vi "Start AC Source.vi"(7 "AC sync source":T1, 8 "error in (no error)":errorcluster, 9 "Signal amplitude (V)":dbl, 10 "Signal frequency  (Hz)":dbl, 11 "AC source":T1) -> (0 "error out":errorcluster, 2 "status":string, 3 "AC source out":T1, 5 "AC sync source out":T1)   [LabVIEW 2020]
doc: "Set required values and properties to the AC source and switch it on."
uses:
  Type definitions/AC Source.ctl
  Type definitions/AC Source type.ctl
  <vilib>/Utility/error.llb/Error Cluster From Error Code.vi
  <vilib>/ErrorRing/Error Ring.xnode
  external libraries/Fluke 5XXX Series Multicalibrator/Fluke 5XXX Series Multicalibrators.lvlib
  external libraries/AWG/AFG3000/Tektronix AFG 3000 Series.lvlib
  external libraries/varilib/varilib.lvlib
  external libraries/AWG/Agilent 33XXX Series/Agilent 33XXX Series.lvlib
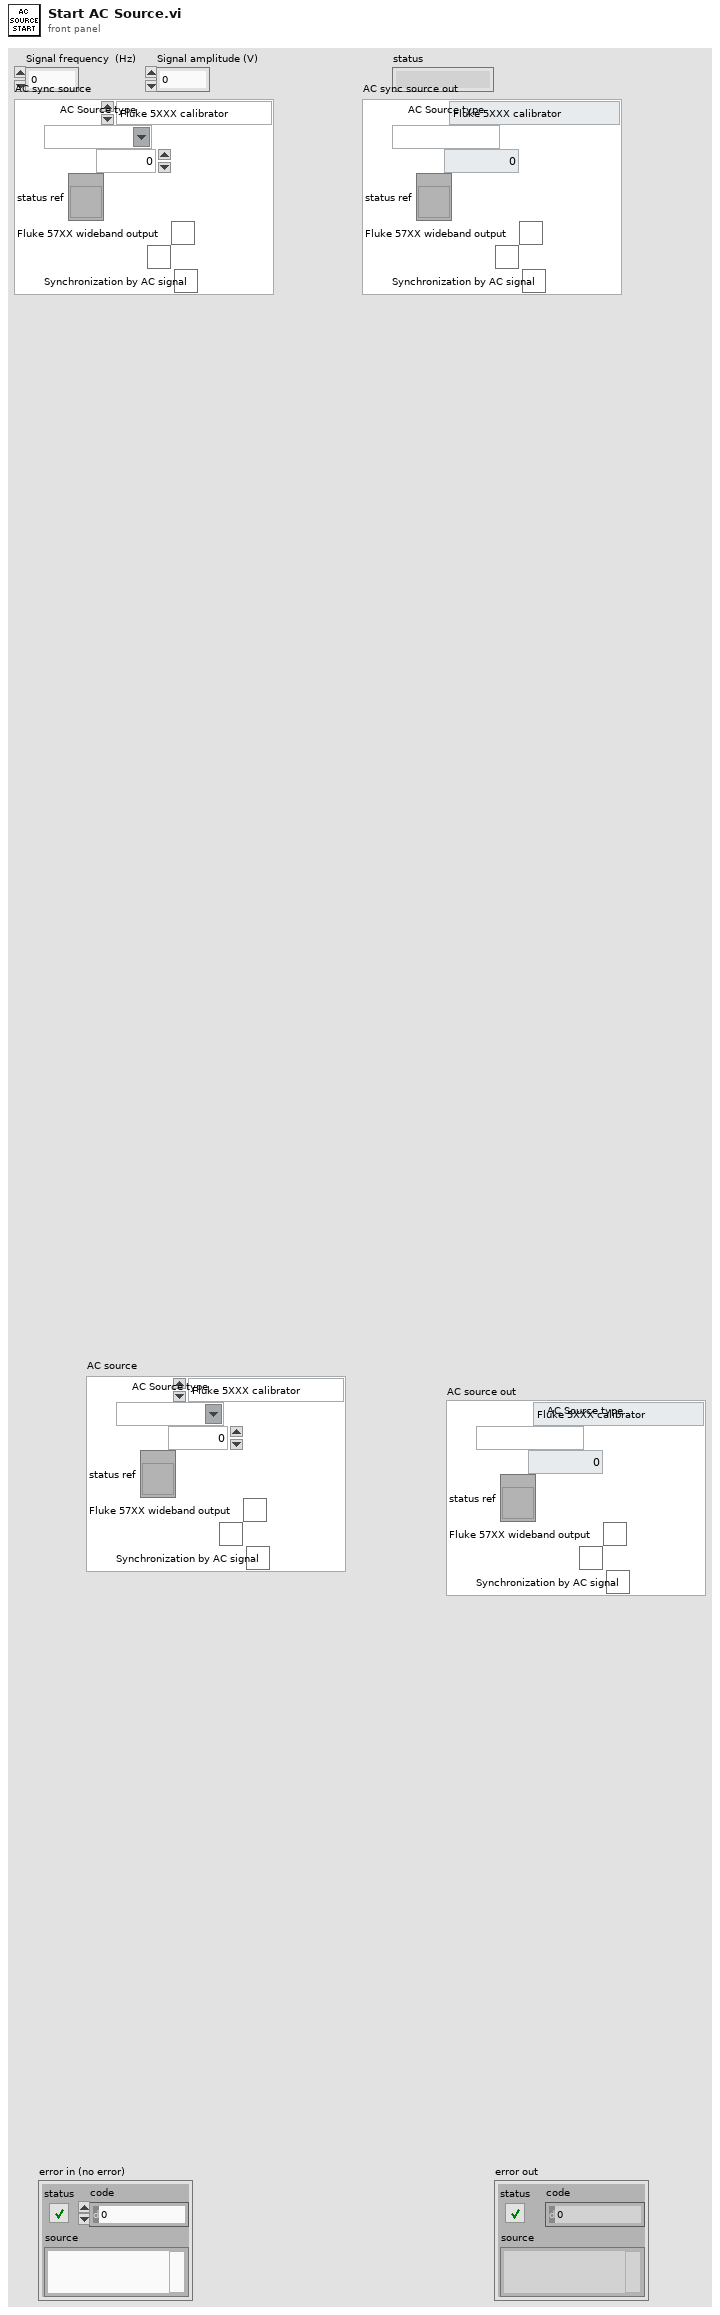
[diagram p1: front panel]
types:
  T1 = typedef "AC Source.ctl" = cluster{"AC Source type":T2, "VISA":refnum<visa-resource-name>, "Ref. clock (Hz)":dbl, "status ref":refnum<vi>, "Fluke 57XX wideband output":bool, "Fluke 57XX ignore errors":bool, "Synchronization by AC signal":bool}
  T2 = typedef "AC Source type.ctl" = enum16{"Fluke 5XXX calibrator", "Tektronix AFG3000 series", "dummy", "Agilent 331xxA to 332xxA", "Agilent 335xxA to 336xxA"}
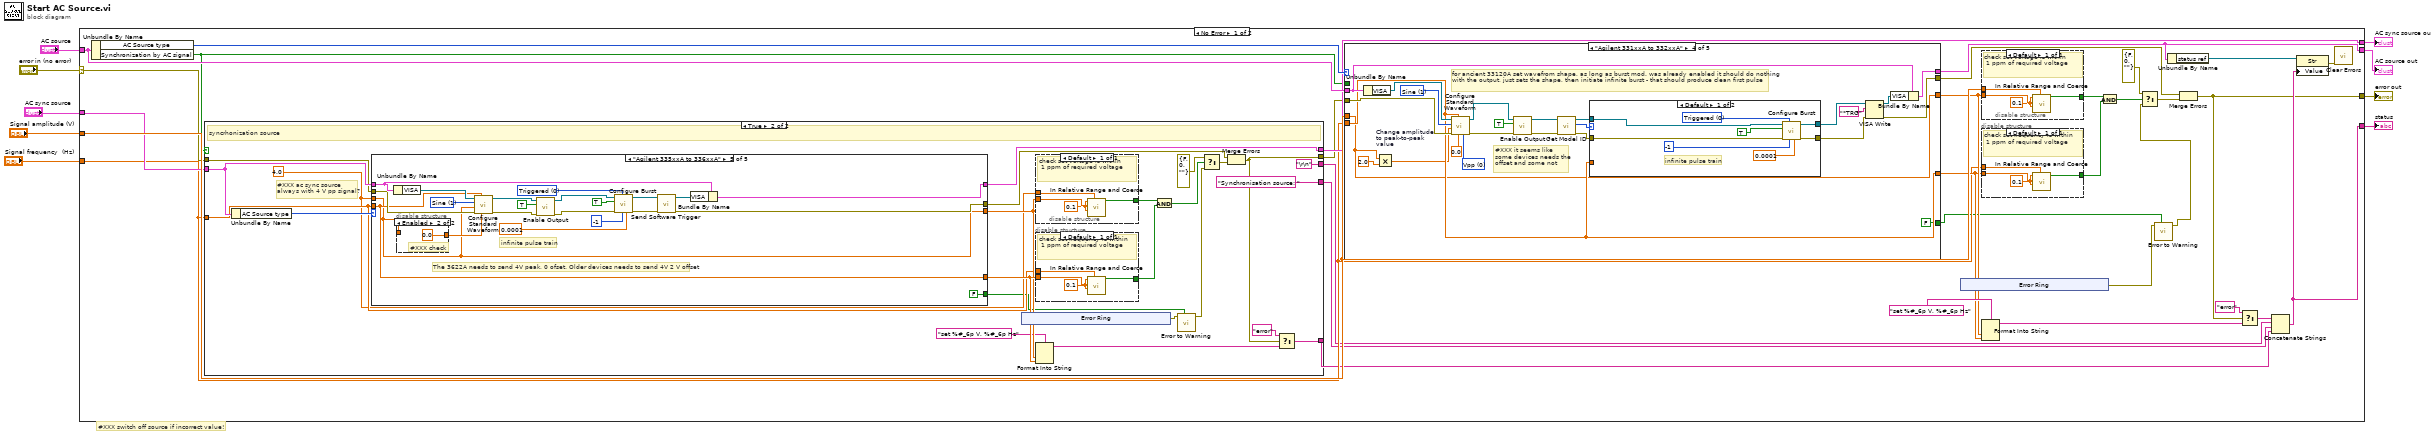
[diagram p0: block diagram]
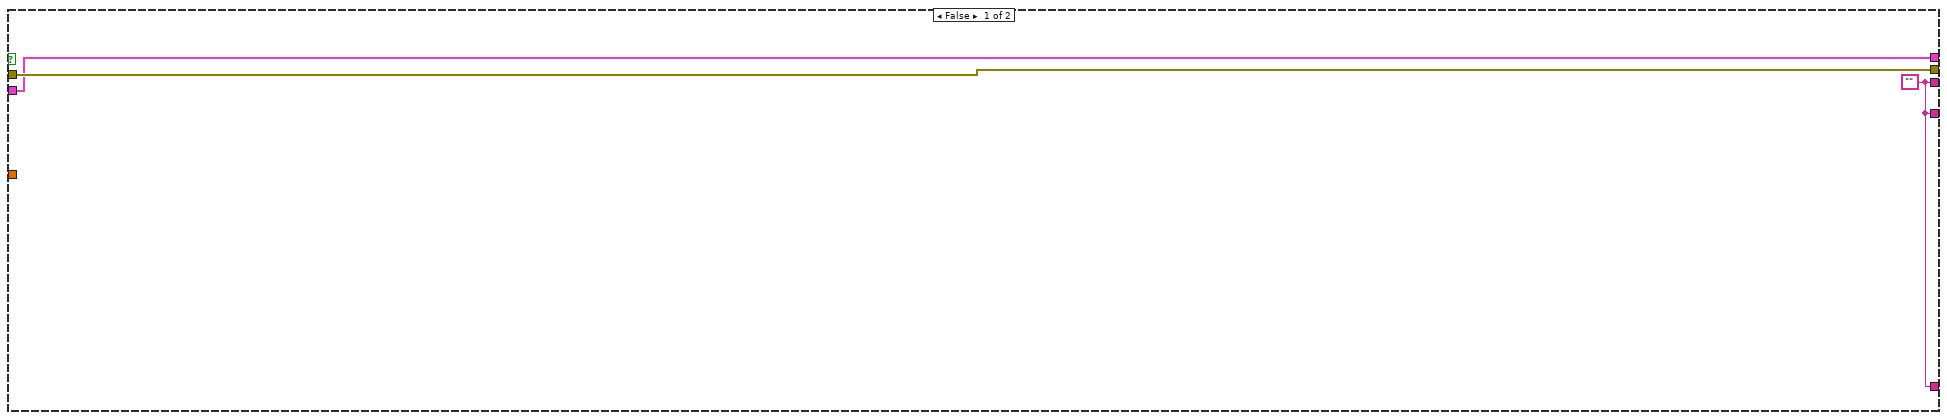
[diagram p2: hidden frame]
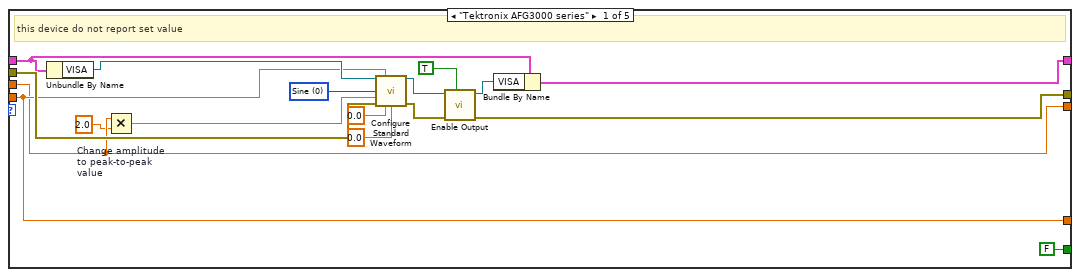
[diagram p3: hidden frame]
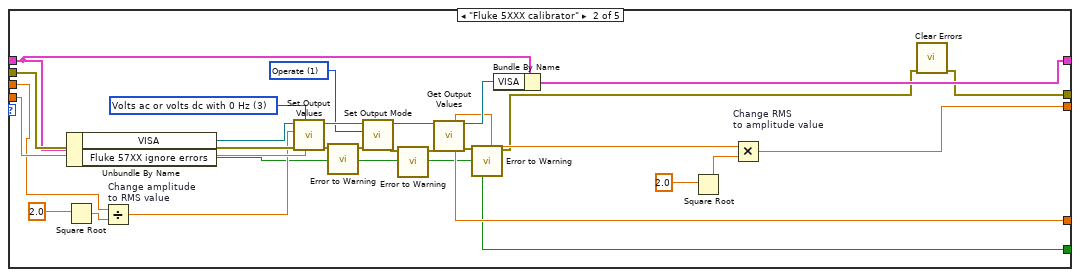
[diagram p4: hidden frame]
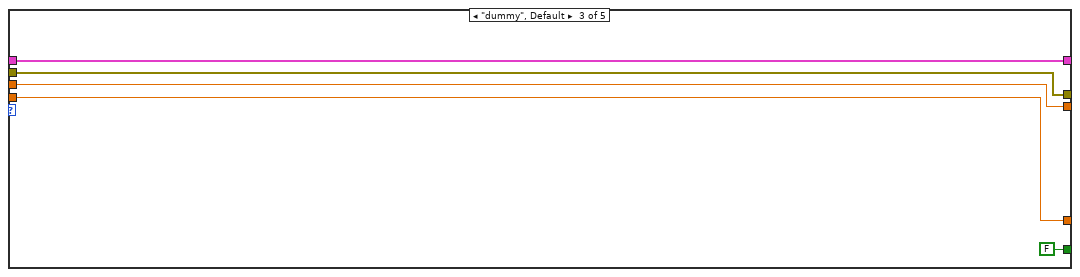
[diagram p5: hidden frame]
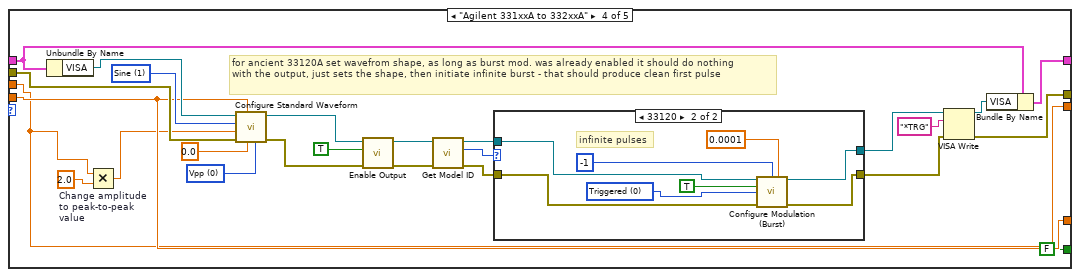
[diagram p6: hidden frame]
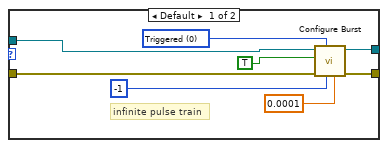
[diagram p7: hidden frame]
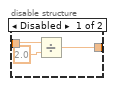
[diagram p8: hidden frame]
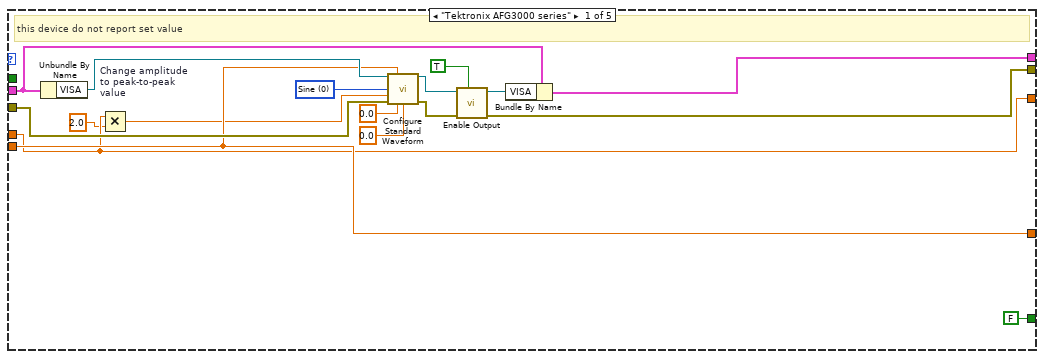
[diagram p9: hidden frame]
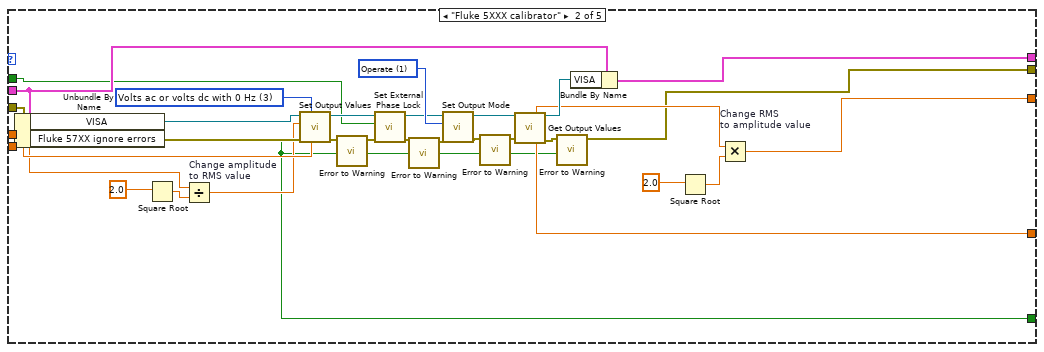
[diagram p10: hidden frame]
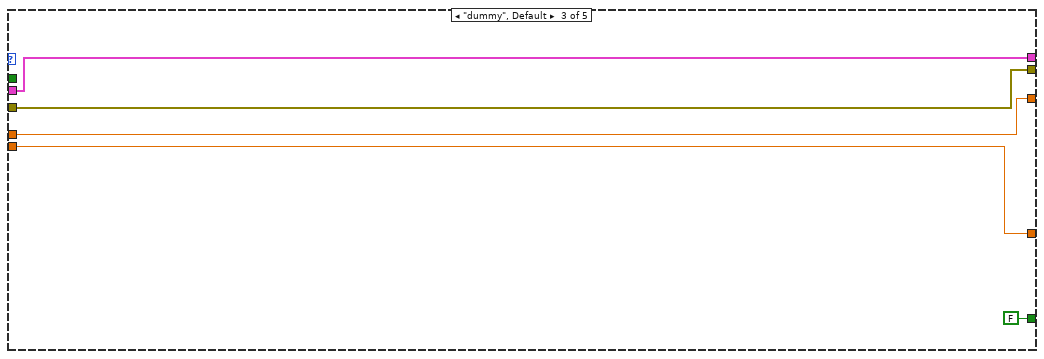
[diagram p11: hidden frame]
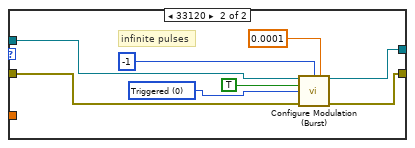
[diagram p12: hidden frame]
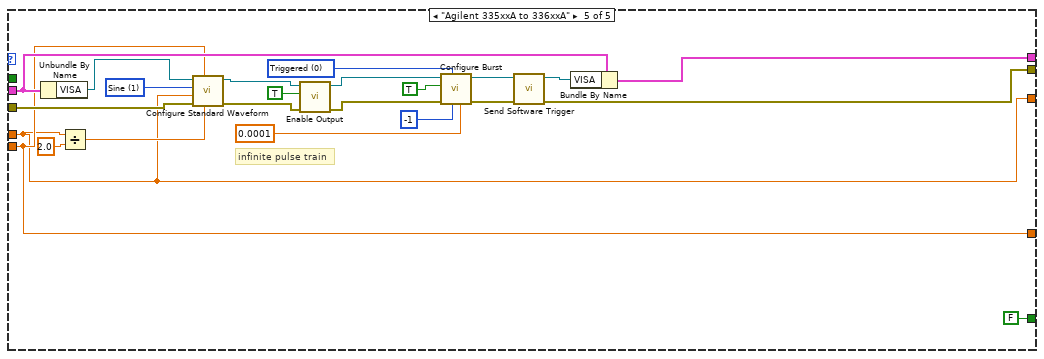
[diagram p13: hidden frame]
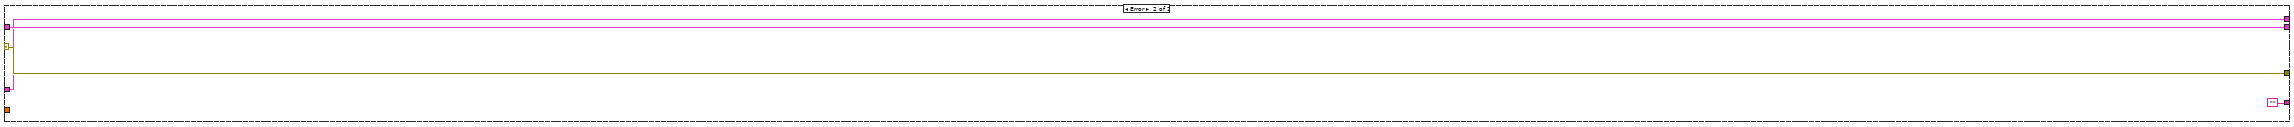
[diagram p14: hidden frame]
diagram:
  # "#XXX switch off source if incorrect value!"
  n1 = case shown="No Error" "error in (no error)" {
    selector: "error in (no error)" -> [w15 w330]
    tunnel: "AC source" -> [w40 w328]
    tunnel: "Signal frequency  (Hz)" -> [w20 _]
    tunnel: "Signal amplitude (V)" -> [w37 _]
    tunnel: [w14 w330] -> w7
    tunnel: [w21 ""] -> w6
    tunnel: [w25 w328] -> w4
    tunnel: "AC sync source" -> [w24 w327]
    tunnel: [w23 w327] -> w2
    frame No Error {
      n2 = Unbundle By Name(w40) -> ("AC Source type"=w41:T2, "Synchronization by AC signal"=w16:bool)
      n3 = case shown="True" w16 {
        tunnel: w15 -> [w44 w57]
        tunnel: [w44 w48] -> w13
        tunnel: w24 -> [w43 w58]
        tunnel: [w43 w56] -> w23
        tunnel: w20 -> [_ w50]
        tunnel: [w42 "\r\n"] -> w19
        tunnel: [w42 "Synchronisation source: " ("string")] -> w18
        tunnel: [w42 w51] -> w17
        frame False {
          w42 = ""
        }
        frame True {
          w49 = 4.0 ("Signal frequency  (Hz)")
          # "#XXX ac sync source\nalways with 4 V pp signal?"
          # "syncrhonization source"
          n4 = Unbundle By Name(w58) -> ("AC Source type"=w59:T2)
          n5 = case shown="\"Agilent 335xxA to 336xxA\"" w59 {
            tunnel: w57 -> [w95 w125 w129 w146 w179]
            tunnel: [w87 w106 w129 w138 w177] -> w66
            tunnel: w58 -> [w93 w124 w130 w144 w181]
            tunnel: [w92 w123 w130 w143 w180] -> w56
            tunnel: w50 -> [w86 w115 w127 w137 w174]
            tunnel: w49 -> [w85 w112 w128 w132 w173]
            tunnel: [w85 w107 w128 w132 w173] -> w63
            tunnel: [w86 w116 w127 w137 w174] -> w64
            tunnel: [FALSE ("Fluke 57XX ignore errors") w99 FALSE ("Fluke 57XX ignore errors") FALSE ("Fluke 57XX ignore errors") FALSE ("Fluke 57XX ignore errors")] -> w45
            frame "Tektronix AFG3000 series" {
              w96 = u16 0 items=["Sine", "Square", "Pulse", "Ramp", "Noise", "DC", "Sin(x)/x", "Gaussian", "Lorentz", "Exponential Rise", "Exponential Decay", "Haversine"] ("Waveform Function (0: Sine)")
              # "this device do not report set value"
              n6 = Unbundle By Name(w93) -> ("VISA"=w94:refnum<visa-resource-name>)
              n7 = Multiply "Change amplitude\nto peak-to-peak\nvalue"(x=w85, y=2.0) -> (x*y=w83:dbl)
              n8 = call "Configure Standard Waveform.vi"("VISA resource name"=w94, "Frequency (1000 Hz)"=w86, "Waveform Function (0: Sine)"=w96, "Amplitude (1 Vpp)"=w83, "error in (no error)"=w95, "DC Offset (0.00 V)"=0.0, "Phase Level (-1)"=0.0) -> ("VISA resource name out"=w90:refnum<visa-resource-name>, "error out"=w88:errorcluster)  [unwired: 7 in]
              n9 = call "Enable Output.vi"("Enable Output (T: Enable)"=TRUE, "error in (no error)"=w88, "VISA resource name"=w90) -> ("error out"=w87:errorcluster, "VISA resource name out"=w89:refnum<visa-resource-name>)  [unwired: 7 in]
              n10 = Bundle By Name(cluster=w93, "VISA"=w89) -> (w92:T1)
            }
            frame "Fluke 5XXX calibrator" {
              w119 = u32 1 items=["Standby", "Operate"] ("Output Mode (0: Standby)")
              w121 = u32 3 items=["Amplitude", "Volts dc or update volts ac", "Volts ac dBm update", "Volts ac or volts dc with 0 Hz", "Volts ac in dBm", "Current dc or update current ac", "Current ac", "Update frequency", "Resistance", "Capacitance", "Temperature (Celsius)", "Temperature (Fahrenheit)", "Power dc or update power ac", "Power ac", "Dual volts dc or update dual ac", "Dual volts ac in volts", "Power ac in dBm update", "Power ac in dBm", "Dual volts ac in dBm update", "Dual volts ac in dBm"] ("Output Value(s) (0 - Amplitude)")
              n11 = Square Root(x=2.0 ("y")) -> (sqrt(x)=w113:dbl)
              n12 = Unbundle By Name(w124) -> ("VISA"=w122:refnum<visa-resource-name>, "Fluke 57XX ignore errors"=w99:bool)
              n13 = Divide "Change amplitude\nto RMS value"(x=w112, y=w113) -> (x/y=w111:dbl)
              n14 = call "Set Output Values.vi"("Fundamental Frequency (0.0 Hz)"=w115, "Output Value(s) (0 - Amplitude)"=w121, "error in (no error)"=w125, "Primary Value (0.0)"=w111, "VISA resource name"=w122) -> ("error out"=w105:errorcluster, "VISA resource name out"=w120:refnum<visa-resource-name>)  [unwired: 5 in]
              n15 = call "Error to Warning.vi"("Change to warning?"=w99, "error in (no error)"=w105) -> ("error out"=w104:errorcluster)  [unwired: 9 in]
              n16 = call "Set Output Mode.vi"("error in (no error)"=w104, "Output Mode (0: Standby)"=w119, "VISA resource name"=w120) -> ("error out"=w103:errorcluster, "VISA resource name out"=w118:refnum<visa-resource-name>)  [unwired: 7 in]
              n17 = call "Error to Warning.vi"("Change to warning?"=w99, "error in (no error)"=w103) -> ("error out"=w102:errorcluster)  [unwired: 9 in]
              n18 = call "Get Output Values.vi"("VISA resource name"=w118, "error in (no error)"=w102) -> ("Primary Value"=w108:dbl, "VISA resource name out"=w117:refnum<visa-resource-name>, "Fundamental Frequency"=w116:dbl, "error out"=w101:errorcluster)  [unwired: 7 in, 3 out]
              n19 = call "Error to Warning.vi"("Change to warning?"=w99, "error in (no error)"=w101) -> ("error out"=w100:errorcluster)  [unwired: 9 in]
              n20 = Bundle By Name(cluster=w124, "VISA"=w117) -> (w123:T1)
              n21 = Square Root(x=2.0 ("y")) -> (sqrt(x)=w110:dbl)
              n22 = Multiply "Change RMS\nto amplitude value"(x=w108, y=w110) -> (x*y=w107:dbl)
              n23 = call <vilib>:"Clear Errors.vi"("error in (no error)"=w100) -> ("error out"=w106:errorcluster)  [unwired: 5 in, 1 out]
            }
            frame "dummy", Default {
            }
            frame "Agilent 331xxA to 332xxA" {
              w136 = u16 0 items=["Vpp", "Vrms", "dB"] ("Unit (0: Vpp)")
              w155 = u16 1 items=["DC", "Sine", "Square", "Triangle", "Ramp", "Pulse", "Noise", "Sinc", "Negative Ramp", "Exponential Rise", "Exponential Fall", "Cardiac"] ("Waveform Function (1: Sine)")
              # "for ancient 33120A set wavefrom shape, as long as burst mod. was already enabled it should do nothing\nwith the output, just sets the shape, then initiate infinite burst - that should produce clean first pulse"
              n24 = Unbundle By Name(w144) -> ("VISA"=w145:refnum<visa-resource-name>)
              n25 = Multiply "Change amplitude\nto peak-to-peak\nvalue"(x=w132, y=2.0) -> (x*y=w131:dbl)
              n26 = call "Configure Standard Waveform.vi"("Unit (0: Vpp)"=w136, "DC Offset (0.00 V)"=0.0, "Frequency (1000 Hz)"=w137, "error in (no error)"=w146, "Amplitude (1)"=w131, "Waveform Function (1: Sine)"=w155, "VISA resource name"=w145) -> ("error out"=w154:errorcluster, "VISA resource name out"=w153:refnum<visa-resource-name>)  [unwired: 3 in]
              n27 = call "Enable Output.vi"("error in (no error)"=w154, "Enable Output  (T: Enable)"=TRUE, "VISA resource name"=w153) -> ("error out"=w151:errorcluster, "VISA resource name out"=w150:refnum<visa-resource-name>)  [unwired: 7 in]
              n28 = call "Get Model ID.vi"("error in (no error)"=w151, "VISA resource name"=w150) -> ("error out"=w149:errorcluster, "model ID"=w148:u32, "VISA resource name out"=w147:refnum<visa-resource-name>)  [unwired: 7 in]
              n29 = case shown="33120" w148 {
                tunnel: [w162 w168] -> w139
                tunnel: [w161 w167] -> w141
                tunnel: w149 -> [w163 w166]
                tunnel: w147 -> [w160 w165]
                frame Default {
                  w159 = u16 0 items=["Triggered", "Gated"] ("Burst Mode (0: Triggered)")
                  # "infinite pulse train"
                  n30 = call "Configure Burst.vi"("Burst Period (1 s)"=0.0001, "Burst Count (1)"=-1, "Burst Mode (0: Triggered)"=w159, "error in (no error)"=w163, "Enable Burst (T: Enable)"=TRUE, "VISA resource name"=w160) -> ("error out"=w162:errorcluster, "VISA resource name out"=w161:refnum<visa-resource-name>)  [unwired: 4 in]
                }
                frame 33120 {
                  w169 = u16 0 items=["Triggered", "Gated"] ("Burst Modulation Mode (0: Triggered)")
                  # "infinite pulses"
                  n31 = call "Configure Modulation (Burst).vi"("VISA resource name"=w165, "Burst Count (1)"=-1, "Burst Period (1 s)"=0.0001, "Enable Burst Modulation (T: Enable)"=TRUE, "Burst Modulation Mode (0: Triggered)"=w169, "error in (no error)"=w166) -> ("VISA resource name out"=w167:refnum<visa-resource-name>, "error out"=w168:errorcluster)  [unwired: 8 in]
                }
              }
              n32 = VISA Write(VISA resource name=w141, write buffer="*TRG", error in (no error)=w139) -> (VISA resource name out=w140:refnum<visa-resource-name>, error out=w138:errorcluster)  [unwired: 1 out]
              n33 = Bundle By Name(cluster=w144, "VISA"=w140) -> (w143:T1)
            }
            frame "Agilent 335xxA to 336xxA" {
              w188 = u16 0 items=["Triggered", "Gated"] ("Burst Mode (0: Triggered)")
              w193 = u16 1 items=["DC", "Sine", "Square", "Triangle", "Ramp", "Pulse", "Noise", "Sinc", "Negative Ramp", "Exponential Rise", "Exponential Fall", "Cardiac"] ("Waveform Function (1: Sine)")
              # "The 3622A needs to send 4V peak, 0 ofset. Older devices needs to send 4V 2 V offset"
              # "infinite pulse train"
              n34 = Unbundle By Name(w181) -> ("VISA"=w189:refnum<visa-resource-name>)
              n35 = disable-structure shown="Enabled" {
                disable-tunnel: [w195 0.0 ("DC Offset (0.00 V)")] -> w182
                disable-tunnel: w173 -> [w194 _]
                frame Disabled {
                  n36 = Divide(x=w194, y=2.0 ("DC Offset (0.00 V)")) -> (x/y=w195:dbl)
                }
                frame Enabled {
                  # "#XXX check"
                }
              }
              n37 = call "Configure Standard Waveform.vi"("DC Offset (0.00 V)"=w182, "Frequency (1000 Hz)"=w174, "error in (no error)"=w179, "Amplitude (1)"=w173, "Waveform Function (1: Sine)"=w193, "VISA resource name"=w189) -> ("error out"=w192:errorcluster, "VISA resource name out"=w191:refnum<visa-resource-name>)  [unwired: 4 in]
              n38 = call "Enable Output.vi"("error in (no error)"=w192, "Enable Output  (T: Enable)"=TRUE, "VISA resource name"=w191) -> ("error out"=w184:errorcluster, "VISA resource name out"=w183:refnum<visa-resource-name>)  [unwired: 7 in]
              n39 = call "Configure Burst.vi"("Burst Period (1 s)"=0.0001, "Burst Count (1)"=-1, "Burst Mode (0: Triggered)"=w188, "error in (no error)"=w184, "Enable Burst (T: Enable)"=TRUE, "VISA resource name"=w183) -> ("error out"=w178:errorcluster, "VISA resource name out"=w176:refnum<visa-resource-name>)  [unwired: 4 in]
              n40 = call "Send Software Trigger.vi"("error in (no error)"=w178, "VISA resource name"=w176) -> ("error out"=w177:errorcluster, "VISA resource name out"=w175:refnum<visa-resource-name>)  [unwired: 8 in]
              n41 = Bundle By Name(cluster=w181, "VISA"=w175) -> (w180:T1)
            }
          }
          n42 = xnode "Error Ring"() -> ("error out"=w47:errorcluster)
          n43 = disable-structure shown="Default" {
            disable-tunnel: w63 -> [w81]
            disable-tunnel: [w80] -> w60
            disable-tunnel: w49 -> [w78]
            frame Enabled {
              w79 = 0.1 ("relative upper limit")
              # "check set voltage is within\n 1 ppm of required voltage"
              n44 = call "In Relative Range and Coerce.vi"("relative base"=w78, "relative lower limit"=w79, "x"=w81, "relative upper limit"=w79) -> ("In Range?"=w80:bool)  [unwired: 6 in, 1 out]
            }
          }
          n45 = disable-structure shown="Default" {
            disable-tunnel: [w77] -> w61
            disable-tunnel: w50 -> [w75]
            disable-tunnel: w64 -> [w74]
            frame Enabled {
              w76 = 0.1 ("relative upper limit")
              # "check set frequency is within\n 1 ppm of required voltage"
              n46 = call "In Relative Range and Coerce.vi"("relative base"=w75, "relative lower limit"=w76, "x"=w74, "relative upper limit"=w76) -> ("In Range?"=w77:bool)  [unwired: 6 in, 1 out]
            }
          }
          n47 = Format Into String(format string="set %#_6p V, %#_6p Hz", w63, w64) -> (resulting string=w52:string)  [unwired: 2 in, 1 out]
          n48 = Compound Arithmetic op=AND(w60, w61) -> (w67:bool)
          n49 = call "Error to Warning.vi"("Change to warning?"=w45, "error in (no error)"=w47) -> ("error out"=w46:errorcluster)  [unwired: 9 in]
          n50 = Select(t=errorcluster {"status"=FALSE, "code"=0, "source"=""}, s=w67, f=w46) -> (s? t:f=w68:errorcluster)
          n51 = Merge Errors(w66, w68) -> (w48:errorcluster)
          n52 = Select(t="error" ("idn string"), s=w48, f=w52) -> (s? t:f=w51:string)
        }
      }
      n53 = case shown="\"Agilent 331xxA to 332xxA\"" w41 {
        tunnel: w13 -> [w224 w257 w261 w278 w311]
        tunnel: [w216 w229 w261 w270 w309] -> w30
        tunnel: w40 -> [w222 w256 w262 w276 w313]
        tunnel: [w221 w255 w262 w275 w312] -> w25
        tunnel: w20 -> [w215 w248 w259 w269 w306]
        tunnel: w37 -> [w214 w242 w260 w264 w305]
        tunnel: [w214 w237 w260 w264 w305] -> w34
        tunnel: [w215 w249 w259 w269 w306] -> w32
        tunnel: w16 -> [_ w245 _ _ _]
        tunnel: [FALSE ("Fluke 57XX ignore errors") w228 FALSE ("Fluke 57XX ignore errors") FALSE ("Fluke 57XX ignore errors") FALSE ("Fluke 57XX ignore errors")] -> w11
        frame "Tektronix AFG3000 series" {
          w225 = u16 0 items=["Sine", "Square", "Pulse", "Ramp", "Noise", "DC", "Sin(x)/x", "Gaussian", "Lorentz", "Exponential Rise", "Exponential Decay", "Haversine"] ("Waveform Function (0: Sine)")
          # "this device do not report set value"
          n54 = Unbundle By Name(w222) -> ("VISA"=w223:refnum<visa-resource-name>)
          n55 = Multiply "Change amplitude\nto peak-to-peak\nvalue"(x=w214, y=2.0) -> (x*y=w212:dbl)
          n56 = call "Configure Standard Waveform.vi"("VISA resource name"=w223, "Frequency (1000 Hz)"=w215, "Waveform Function (0: Sine)"=w225, "Amplitude (1 Vpp)"=w212, "error in (no error)"=w224, "DC Offset (0.00 V)"=0.0, "Phase Level (-1)"=0.0) -> ("VISA resource name out"=w219:refnum<visa-resource-name>, "error out"=w217:errorcluster)  [unwired: 7 in]
          n57 = call "Enable Output.vi"("Enable Output (T: Enable)"=TRUE, "error in (no error)"=w217, "VISA resource name"=w219) -> ("error out"=w216:errorcluster, "VISA resource name out"=w218:refnum<visa-resource-name>)  [unwired: 7 in]
          n58 = Bundle By Name(cluster=w222, "VISA"=w218) -> (w221:T1)
        }
        frame "Fluke 5XXX calibrator" {
          w252 = u32 1 items=["Standby", "Operate"] ("Output Mode (0: Standby)")
          w253 = u32 3 items=["Amplitude", "Volts dc or update volts ac", "Volts ac dBm update", "Volts ac or volts dc with 0 Hz", "Volts ac in dBm", "Current dc or update current ac", "Current ac", "Update frequency", "Resistance", "Capacitance", "Temperature (Celsius)", "Temperature (Fahrenheit)", "Power dc or update power ac", "Power ac", "Dual volts dc or update dual ac", "Dual volts ac in volts", "Power ac in dBm update", "Power ac in dBm", "Dual volts ac in dBm update", "Dual volts ac in dBm"] ("Output Value(s) (0 - Amplitude)")
          n59 = Unbundle By Name(w256) -> ("VISA"=w254:refnum<visa-resource-name>, "Fluke 57XX ignore errors"=w228:bool)
          n60 = Square Root(x=2.0 ("y")) -> (sqrt(x)=w244:dbl)
          n61 = Divide "Change amplitude\nto RMS value"(x=w242, y=w244) -> (x/y=w241:dbl)
          n62 = call "Set Output Values.vi"("Fundamental Frequency (0.0 Hz)"=w248, "Output Value(s) (0 - Amplitude)"=w253, "error in (no error)"=w257, "Primary Value (0.0)"=w241, "VISA resource name"=w254) -> ("error out"=w236:errorcluster, "VISA resource name out"=w246:refnum<visa-resource-name>)  [unwired: 5 in]
          n63 = call "Error to Warning.vi"("Change to warning?"=w228, "error in (no error)"=w236) -> ("error out"=w235:errorcluster)  [unwired: 9 in]
          n64 = call "Set External Phase Lock.vi"("error in (no error)"=w235, "External Phase Lock (F: Off)"=w245, "VISA resource name"=w246) -> ("error out"=w234:errorcluster, "VISA resource name out"=w247:refnum<visa-resource-name>)  [unwired: 7 in]
          n65 = call "Error to Warning.vi"("Change to warning?"=w228, "error in (no error)"=w234) -> ("error out"=w233:errorcluster)  [unwired: 9 in]
          n66 = call "Set Output Mode.vi"("error in (no error)"=w233, "Output Mode (0: Standby)"=w252, "VISA resource name"=w247) -> ("error out"=w232:errorcluster, "VISA resource name out"=w251:refnum<visa-resource-name>)  [unwired: 7 in]
          n67 = call "Error to Warning.vi"("Change to warning?"=w228, "error in (no error)"=w232) -> ("error out"=w231:errorcluster)  [unwired: 9 in]
          n68 = call "Get Output Values.vi"("VISA resource name"=w251, "error in (no error)"=w231) -> ("Primary Value"=w238:dbl, "VISA resource name out"=w250:refnum<visa-resource-name>, "Fundamental Frequency"=w249:dbl, "error out"=w230:errorcluster)  [unwired: 7 in, 3 out]
          n69 = call "Error to Warning.vi"("Change to warning?"=w228, "error in (no error)"=w230) -> ("error out"=w229:errorcluster)  [unwired: 9 in]
          n70 = Bundle By Name(cluster=w256, "VISA"=w250) -> (w255:T1)
          n71 = Square Root(x=2.0 ("y")) -> (sqrt(x)=w239:dbl)
          n72 = Multiply "Change RMS\nto amplitude value"(x=w238, y=w239) -> (x*y=w237:dbl)
        }
        frame "dummy", Default {
        }
        frame "Agilent 331xxA to 332xxA" {
          w266 = u16 0 items=["Vpp", "Vrms", "dB"] ("Unit (0: Vpp)")
          w287 = u16 1 items=["DC", "Sine", "Square", "Triangle", "Ramp", "Pulse", "Noise", "Sinc", "Negative Ramp", "Exponential Rise", "Exponential Fall", "Cardiac"] ("Waveform Function (1: Sine)")
          # "#XXX it seems like\nsome devices needs the\noffset and some not"
          # "for ancient 33120A set wavefrom shape, as long as burst mod. was already enabled it should do nothing\nwith the output, just sets the shape, then initiate infinite burst - that should produce clean first pulse"
          n73 = Unbundle By Name(w276) -> ("VISA"=w277:refnum<visa-resource-name>)
          n74 = Multiply "Change amplitude\nto peak-to-peak\nvalue"(x=w264, y=2.0) -> (x*y=w263:dbl)
          n75 = call "Configure Standard Waveform.vi"("Unit (0: Vpp)"=w266, "DC Offset (0.00 V)"=0.0, "Frequency (1000 Hz)"=w269, "error in (no error)"=w278, "Amplitude (1)"=w263, "Waveform Function (1: Sine)"=w287, "VISA resource name"=w277) -> ("error out"=w286:errorcluster, "VISA resource name out"=w285:refnum<visa-resource-name>)  [unwired: 3 in]
          n76 = call "Enable Output.vi"("error in (no error)"=w286, "Enable Output  (T: Enable)"=TRUE, "VISA resource name"=w285) -> ("error out"=w283:errorcluster, "VISA resource name out"=w282:refnum<visa-resource-name>)  [unwired: 7 in]
          n77 = call "Get Model ID.vi"("error in (no error)"=w283, "VISA resource name"=w282) -> ("error out"=w281:errorcluster, "model ID"=w280:u32, "VISA resource name out"=w279:refnum<visa-resource-name>)  [unwired: 7 in]
          n78 = case shown="Default" w280 {
            tunnel: [w294 w300] -> w271
            tunnel: [w293 w299] -> w273
            tunnel: w269 -> [_ _]
            tunnel: w281 -> [w295 w298]
            tunnel: w279 -> [w292 w297]
            frame Default {
              w291 = u16 0 items=["Triggered", "Gated"] ("Burst Mode (0: Triggered)")
              # "infinite pulse train"
              n79 = call "Configure Burst.vi"("Burst Period (1 s)"=0.0001, "Burst Count (1)"=-1, "Burst Mode (0: Triggered)"=w291, "error in (no error)"=w295, "Enable Burst (T: Enable)"=TRUE, "VISA resource name"=w292) -> ("error out"=w294:errorcluster, "VISA resource name out"=w293:refnum<visa-resource-name>)  [unwired: 4 in]
            }
            frame 33120 {
              w301 = u16 0 items=["Triggered", "Gated"] ("Burst Modulation Mode (0: Triggered)")
              # "infinite pulses"
              n80 = call "Configure Modulation (Burst).vi"("VISA resource name"=w297, "Burst Count (1)"=-1, "Burst Period (1 s)"=0.0001, "Enable Burst Modulation (T: Enable)"=TRUE, "Burst Modulation Mode (0: Triggered)"=w301, "error in (no error)"=w298) -> ("VISA resource name out"=w299:refnum<visa-resource-name>, "error out"=w300:errorcluster)  [unwired: 8 in]
            }
          }
          n81 = VISA Write(VISA resource name=w273, write buffer="*TRG", error in (no error)=w271) -> (VISA resource name out=w272:refnum<visa-resource-name>, error out=w270:errorcluster)  [unwired: 1 out]
          n82 = Bundle By Name(cluster=w276, "VISA"=w272) -> (w275:T1)
        }
        frame "Agilent 335xxA to 336xxA" {
          w321 = u16 0 items=["Triggered", "Gated"] ("Burst Mode (0: Triggered)")
          w326 = u16 1 items=["DC", "Sine", "Square", "Triangle", "Ramp", "Pulse", "Noise", "Sinc", "Negative Ramp", "Exponential Rise", "Exponential Fall", "Cardiac"] ("Waveform Function (1: Sine)")
          # "infinite pulse train"
          n83 = Unbundle By Name(w313) -> ("VISA"=w322:refnum<visa-resource-name>)
          n84 = Divide(x=w305, y=2.0 ("DC Offset (0.00 V)")) -> (x/y=w314:dbl)
          n85 = call "Configure Standard Waveform.vi"("DC Offset (0.00 V)"=w314, "Frequency (1000 Hz)"=w306, "error in (no error)"=w311, "Amplitude (1)"=w305, "Waveform Function (1: Sine)"=w326, "VISA resource name"=w322) -> ("error out"=w325:errorcluster, "VISA resource name out"=w324:refnum<visa-resource-name>)  [unwired: 4 in]
          n86 = call "Enable Output.vi"("error in (no error)"=w325, "Enable Output  (T: Enable)"=TRUE, "VISA resource name"=w324) -> ("error out"=w317:errorcluster, "VISA resource name out"=w316:refnum<visa-resource-name>)  [unwired: 7 in]
          n87 = call "Configure Burst.vi"("Burst Period (1 s)"=0.0001, "Burst Count (1)"=-1, "Burst Mode (0: Triggered)"=w321, "error in (no error)"=w317, "Enable Burst (T: Enable)"=TRUE, "VISA resource name"=w316) -> ("error out"=w310:errorcluster, "VISA resource name out"=w308:refnum<visa-resource-name>)  [unwired: 4 in]
          n88 = call "Send Software Trigger.vi"("error in (no error)"=w310, "VISA resource name"=w308) -> ("error out"=w309:errorcluster, "VISA resource name out"=w307:refnum<visa-resource-name>)  [unwired: 8 in]
          n89 = Bundle By Name(cluster=w313, "VISA"=w307) -> (w312:T1)
        }
      }
      n90 = xnode "Error Ring"() -> ("error out"=w10:errorcluster)
      n91 = disable-structure shown="Default" {
        disable-tunnel: w34 -> [w210]
        disable-tunnel: [w209] -> w39
        disable-tunnel: w37 -> [w207]
        frame Enabled {
          w208 = 0.1 ("relative upper limit")
          # "check set voltage is within\n 1 ppm of required voltage"
          n92 = call "In Relative Range and Coerce.vi"("relative base"=w207, "relative lower limit"=w208, "x"=w210, "relative upper limit"=w208) -> ("In Range?"=w209:bool)  [unwired: 6 in, 1 out]
        }
      }
      n93 = disable-structure shown="Default" {
        disable-tunnel: [w206] -> w38
        disable-tunnel: w20 -> [w204]
        disable-tunnel: w32 -> [w203]
        frame Enabled {
          w205 = 0.1 ("relative upper limit")
          # "check set frequency is within\n 1 ppm of required voltage"
          n94 = call "In Relative Range and Coerce.vi"("relative base"=w204, "relative lower limit"=w205, "x"=w203, "relative upper limit"=w205) -> ("In Range?"=w206:bool)  [unwired: 6 in, 1 out]
        }
      }
      n95 = Format Into String(format string="set %#_6p V, %#_6p Hz", w34, w32) -> (resulting string=w36:string)  [unwired: 2 in, 1 out]
      n96 = Compound Arithmetic op=AND(w39, w38) -> (w29:bool)
      n97 = call "Error to Warning.vi"("Change to warning?"=w11, "error in (no error)"=w10) -> ("error out"=w12:errorcluster)  [unwired: 9 in]
      n98 = Select(t=errorcluster {"status"=FALSE, "code"=0, "source"=""}, s=w29, f=w12) -> (s? t:f=w28:errorcluster)
      n99 = Unbundle By Name(w25) -> ("status ref"=w27:refnum<vi>)
      n100 = Merge Errors(w30, w28) -> (w14:errorcluster)
      n101 = Select(t="error" ("idn string"), s=w14, f=w36) -> (s? t:f=w22:string)
      n102 = Concatenate Strings(w22, w19, w18, w17) -> (w21:string)
      n103 = property class="Str"(reference=w27, "Value"=w21) -> (error out=w26:errorcluster)  [unwired: 1 in, 1 out]
      n104 = call <vilib>:"Clear Errors.vi"("error in (no error)"=w26) -> ()  [unwired: 5 in, 2 out]
    }
    frame Error {
    }
  }
  "error out" <- w7
  "status" <- w6
  "AC source out" <- w4
  "AC sync source out" <- w2
